vi "test_CCDSetAndGetXAxisConversionType.vi"(6 "Delay between send and receive [ms]":i32=100, 7 "Test should pass":bool=TRUE, 8 "error in":errorcluster, 9 "tear down connection":bool=TRUE, 10 "set-up a connection":bool=TRUE, 11 "device selection":enum16{"monochromator", "CCD", "SCD"}(ring)=enum."CCD") -> (0 "error out":errorcluster)   [LabVIEW 2023]
uses:
  Classes/CCD/CCD.lvclass
  <vilib>/addons/_JKI Toolkits/Caraya/classes/Assert/Assert Equal Value and Type_Variant.vi
  <vilib>/addons/_JKI Toolkits/Caraya/classes/Assert/Assert Not Error.vi
  <vilib>/addons/_JKI Toolkits/Caraya/classes/Test/Test.lvclass
  <vilib>/addons/_JKI Toolkits/Caraya/classes/Assert/Assert.lvclass
  C:/Users/grju/Desktop/AbgelegteDokumente/Kunden/Horiba/horiba-labview-sdk/Source/Classes/GenericDevice/GenericDevice.lvclass
  C:/Users/grju/Desktop/AbgelegteDokumente/Kunden/Horiba/horiba-labview-sdk/Source/Classes/CCD/CCD.lvclass
panel:
  # "Connector Pane"
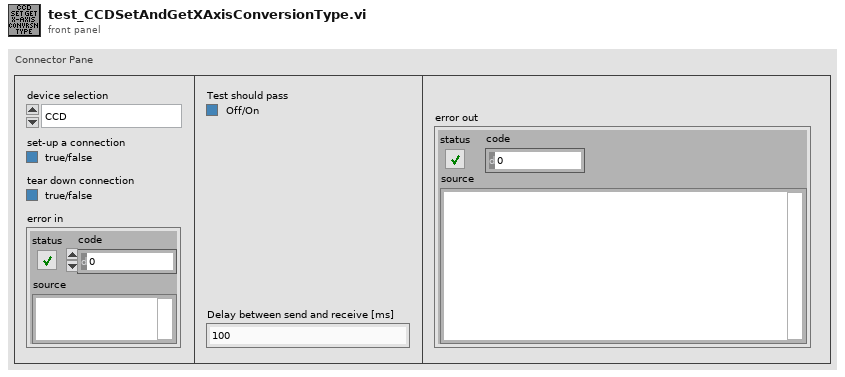
[diagram p1: front panel]
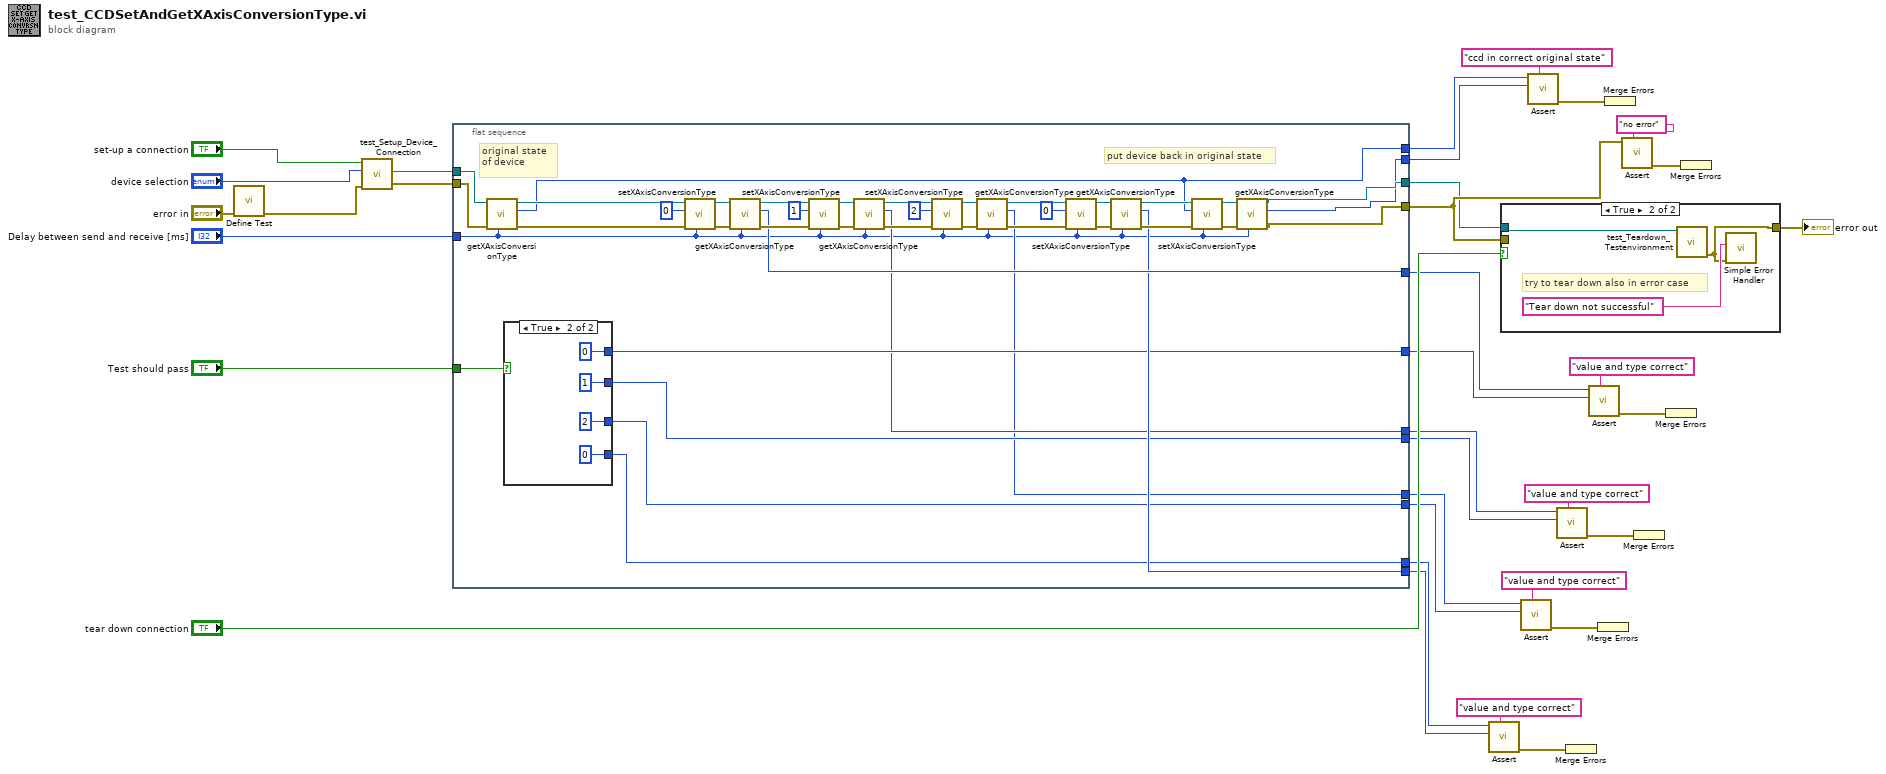
[diagram p0: block diagram]
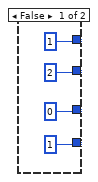
[diagram p2: hidden frame]
diagram:
  n1 = call <vilib>:"Define Test.vi"("error in (no error)"="error in") -> ("error out"=w5:errorcluster)  [unwired: 9 in, 1 out]
  n2 = call "test_Setup_Device_Connection.vi"("error in (no error)"=w5, "device selection"="device selection", "set-up a connection"="set-up a connection") -> ("error out"=w6:errorcluster, "CCD.lvclass"=w4:refnum<class "CCD.lvclass">)  [unwired: 5 in, 2 out]
  n3 = flat-sequence {
    tunnel: w6 -> [w72]
    tunnel: w4 -> [w73]
    tunnel: [w50] -> w27
    tunnel: "Test should pass" -> [w74]
    tunnel: [w49] -> w26
    tunnel: [w48] -> w23
    tunnel: [w51] -> w22
    tunnel: [w47] -> w21
    tunnel: [w44] -> w19
    tunnel: [w40] -> w17
    tunnel: [w46] -> w14
    tunnel: [w45] -> w20
    tunnel: [w43] -> w18
    tunnel: [w41] -> w16
    tunnel: [w42] -> w15
    tunnel: "Delay between send and receive [ms]" -> [w39]
    frame #0 {
      # "put device back in original state"
      # "original state of device"
      n4 = call "getXAxisConversionType.vi"("Delay between send and receive [ms]"=w39, "error in (no error)"=w72, "CCD in"=w73) -> ("error out"=w52:errorcluster, "type"=w51:i32, "CCD out"=w53:refnum<class "CCD.lvclass">)  [unwired: 6 in]
      n5 = case shown="True" w74 {
        tunnel: [1 ("token") 0 ("token")] -> w45
        tunnel: [2 ("token") 1 ("token")] -> w43
        tunnel: [0 ("token") 2 ("token")] -> w41
        tunnel: [1 ("token") 0 ("token")] -> w42
        frame False {
        }
        frame True {
        }
      }
      n6 = call "setXAxisConversionType.vi"("Delay between send and receive [ms]"=w39, "error in (no error)"=w52, "type"=0 ("token"), "CCD in"=w53) -> ("error out"=w61:errorcluster, "CCD out"=w60:refnum<class "CCD.lvclass">)  [unwired: 4 in, 2 out]
      n7 = call "getXAxisConversionType.vi"("Delay between send and receive [ms]"=w39, "error in (no error)"=w61, "CCD in"=w60) -> ("error out"=w65:errorcluster, "type"=w47:i32, "CCD out"=w64:refnum<class "CCD.lvclass">)  [unwired: 6 in]
      n8 = call "setXAxisConversionType.vi"("Delay between send and receive [ms]"=w39, "error in (no error)"=w65, "type"=1 ("token"), "CCD in"=w64) -> ("error out"=w62:errorcluster, "CCD out"=w63:refnum<class "CCD.lvclass">)  [unwired: 4 in, 2 out]
      n9 = call "getXAxisConversionType.vi"("Delay between send and receive [ms]"=w39, "error in (no error)"=w62, "CCD in"=w63) -> ("error out"=w67:errorcluster, "type"=w44:i32, "CCD out"=w66:refnum<class "CCD.lvclass">)  [unwired: 6 in]
      n10 = call "setXAxisConversionType.vi"("Delay between send and receive [ms]"=w39, "error in (no error)"=w67, "type"=2 ("token"), "CCD in"=w66) -> ("error out"=w55:errorcluster, "CCD out"=w54:refnum<class "CCD.lvclass">)  [unwired: 4 in, 2 out]
      n11 = call "getXAxisConversionType.vi"("Delay between send and receive [ms]"=w39, "error in (no error)"=w55, "CCD in"=w54) -> ("error out"=w59:errorcluster, "type"=w40:i32, "CCD out"=w58:refnum<class "CCD.lvclass">)  [unwired: 6 in]
      n12 = call "setXAxisConversionType.vi"("Delay between send and receive [ms]"=w39, "error in (no error)"=w59, "type"=0 ("token"), "CCD in"=w58) -> ("error out"=w56:errorcluster, "CCD out"=w57:refnum<class "CCD.lvclass">)  [unwired: 4 in, 2 out]
      n13 = call "getXAxisConversionType.vi"("Delay between send and receive [ms]"=w39, "error in (no error)"=w56, "CCD in"=w57) -> ("error out"=w71:errorcluster, "type"=w46:i32, "CCD out"=w70:refnum<class "CCD.lvclass">)  [unwired: 6 in]
      n14 = call "setXAxisConversionType.vi"("Delay between send and receive [ms]"=w39, "error in (no error)"=w71, "type"=w51, "CCD in"=w70) -> ("error out"=w68:errorcluster, "CCD out"=w69:refnum<class "CCD.lvclass">)  [unwired: 4 in, 2 out]
      n15 = call "getXAxisConversionType.vi"("Delay between send and receive [ms]"=w39, "error in (no error)"=w68, "CCD in"=w69) -> ("error out"=w50:errorcluster, "type"=w48:i32, "CCD out"=w49:refnum<class "CCD.lvclass">)  [unwired: 6 in]
    }
  }
  n16 = call-poly <vilib>:"Assert.vi"("Label"="value and type correct" ("Label (VI Title)"), "Y"=w14, "X"=w15) -> ("error out"=w33:errorcluster)  [unwired: 7 in, 1 out]
  n17 = case shown="True" "tear down connection" {
    tunnel: w26 -> [_ w85]
    tunnel: [w83 w84] -> w7
    tunnel: w27 -> [w83 _]
    frame False {
    }
    frame True {
      # "try to tear down also in error case"
      n18 = call "test_Teardown_Testenvironment.vi"("GenericDevice.lvclass"=w85) -> ("error out"=w84:errorcluster)  [unwired: 9 in, 1 out]
      n19 = call <vilib>:"Simple Error Handler.vi"("error source (\" \")"="Tear down not successful" ("error source (\" \")"), "error in (no error)"=w84) -> ()  [unwired: 3 in, 5 out]
    }
  }
  "error out" <- w7
  n20 = call-poly <vilib>:"Assert.vi"("Label"="value and type correct" ("Label (VI Title)"), "Y"=w16, "X"=w17) -> ("error out"=w13:errorcluster)  [unwired: 7 in, 1 out]
  n21 = call-poly <vilib>:"Assert.vi"("Label"="ccd in correct original state" ("Label (VI Title)"), "Y"=w23, "X"=w22) -> ("error out"=w25:errorcluster)  [unwired: 7 in, 1 out]
  n22 = call-poly <vilib>:"Assert.vi"("Label"="value and type correct" ("Label (VI Title)"), "Y"=w18, "X"=w19) -> ("error out"=w9:errorcluster)  [unwired: 7 in, 1 out]
  n23 = Merge Errors(w33) -> ()  [unwired: 1 out]
  n24 = call-poly <vilib>:"Assert.vi"("Label"="value and type correct" ("Label (VI Title)"), "Y"=w20, "X"=w21) -> ("error out"=w10:errorcluster)  [unwired: 7 in, 1 out]
  n25 = Merge Errors(w13) -> ()  [unwired: 1 out]
  n26 = Merge Errors(w25) -> ()  [unwired: 1 out]
  n27 = call-poly <vilib>:"Assert.vi"("Label"="no error" ("Label (VI Title)"), "Not Error?"=w27) -> ("error out"=w29:errorcluster)  [unwired: 8 in, 1 out]
  n28 = Merge Errors(w9) -> ()  [unwired: 1 out]
  n29 = Merge Errors(w10) -> ()  [unwired: 1 out]
  n30 = Merge Errors(w29) -> ()  [unwired: 1 out]
